vi "SHA3-384.vi"() -> (0 "Hash Function out":refnum<class "NI_SHA-3.lvclass">)   [LabVIEW 2020, in "NI_SHA-3.lvclass"]
doc: "Returns an instance of the SHA3-384 hash function."
uses:
  <vilib>/security/Message Digest/SHA-3/NI_SHA-3.lvclass
  <vilib>/security/Message Digest/SHA-3/NI_SHA-3.lvclass/NI_SHA-3.ctl
  <vilib>/security/Message Digest/SHA-3/subVIs/SHA-3 Number of Rounds.vi/de10eb19-ecc6-40a5-873c-159babf1c20e.vi
  <vilib>/security/Message Digest/SHA-3/subVIs/Get Word Type.vi
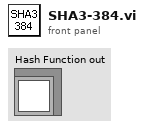
[diagram p1: front panel]
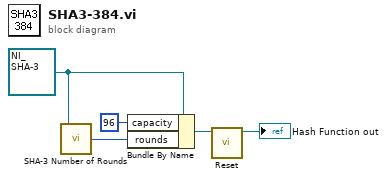
[diagram p0: block diagram]
diagram:
  w1 = refnum<class "NI_SHA-3.lvclass"> refnum ("nihash.lvlib:Keccak-f-1600.lvclass")
  n1 = call <vilib>:"SHA-3 Number of Rounds.vi"("Hash Function in"=w1) -> ("rounds"=w2:i32)
  n2 = Bundle By Name(cluster=w1, "capacity"=96, "rounds"=w2) -> (w4:refnum<class "NI_SHA-3.lvclass">)
  n3 = call <vilib>:"Reset.vi"("Hash Function in"=w4) -> ("Hash Function out"=→"Hash Function out":refnum<class "NI_SHA-3.lvclass">)  [unwired: 10 in]
